vi "websocket initialization handshake.vi"(8 "error in":errorcluster, 11 "upgrade data":T1) -> (0 "error out":errorcluster, 3 "TCP Network Connection out":refnum<k5>)   [LabVIEW 2016, in "websocket upgrade handler.lvclass"]
uses:
  websocket upgrade handler.lvclass
  HTTP responder/http upgrade data.ctl
  HTTP server/http request.ctl
  HTTP server/http method.ctl
  HTTP server/http header data.ctl
  HTTP server/http response.ctl
  HTTP server/http response packet type.ctl
  HTTP server/http add header to set.vi
  HTTP server/Basic HTTP server.lvclass
  websocket core.lvlib
  HTTP server/headers/http headers.lvlib
  HTTP responder/http responder.lvclass
panel:
  out "subprotocol":string
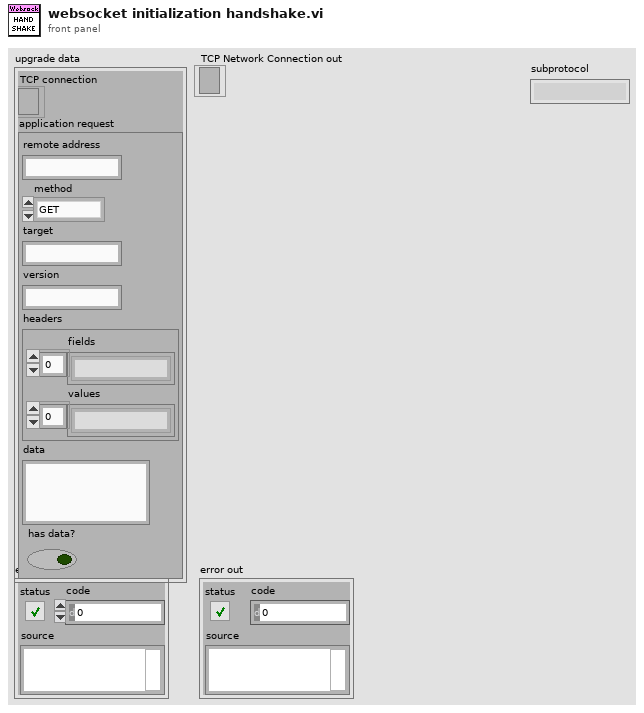
[diagram p1: front panel]
types:
  T1 = typedef "http responder.lvclass/http upgrade data.ctl" = cluster{"TCP connection":refnum<k5>, "application request":T2}
  T2 = typedef "Basic HTTP server.lvclass/http request.ctl" = cluster{"remote address":string, "method":T3, "target":string, "version":string, "headers":T4, "data":string, "has data?":bool}
  T3 = typedef "Basic HTTP server.lvclass/http method.ctl" = enum16{"GET", "POST", "PUT", "DELETE", "HEAD", "OPTIONS", "upgrade"}
  T4 = typedef "http headers.lvlib/http header data.ctl" = cluster{"fields":string[], "values":string[]}
  T5 = typedef "Basic HTTP server.lvclass/http response packet type.ctl" = enum16{"full response", "header only", "data only", "last data"}
  T6 = typedef "Basic HTTP server.lvclass/http response.ctl" = cluster{"packet type":T5, "reason code":u16, "status string":string, "headers":T4, "cookies":string[], "data":string}
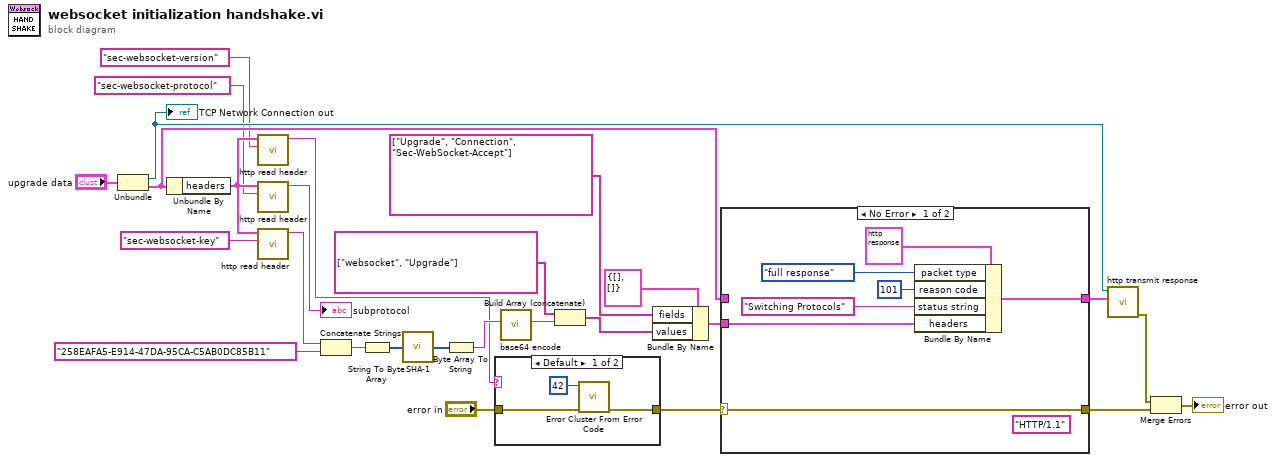
[diagram p0: block diagram]
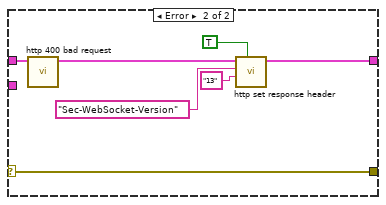
[diagram p3: hidden frame]
diagram:
  n1 = Unbundle("upgrade data") -> ("TCP connection"=w26:refnum<k5>, "application request"=w25:T2)
  "TCP Network Connection out" <- w26
  n2 = Unbundle By Name(w25) -> ("headers"=w8:T4)
  n3 = call "http read header.vi"("header field name"="sec-websocket-version" ("name"), "headers"=w8) -> ("value"=w4:string)  [unwired: 8 in, 1 out]
  n4 = call "http read header.vi"("header field name"="sec-websocket-protocol" ("name"), "headers"=w8) -> ("value"=→"subprotocol":string)  [unwired: 8 in, 1 out]
  n5 = call "http read header.vi"("header field name"="sec-websocket-key" ("name"), "headers"=w8) -> ("value"=w6:string)  [unwired: 8 in, 1 out]
  n6 = Concatenate Strings(w6, "258EAFA5-E914-47DA-95CA-C5AB0DC85B11") -> (w18:string)
  n7 = String To Byte Array(string=w18) -> (unsigned byte array=w17:u8[])
  n8 = call "SHA-1.vi"("Data"=w17) -> ("message-digest"=w16:u8[])
  n9 = Byte Array To String(unsigned byte array=w16) -> (string=w15:string)
  n10 = case shown="Default" w4 {
    tunnel: [w29 w31] -> w20
    tunnel: "error in" -> [w30 w31]
    frame Default {
      n11 = call <vilib>:"Error Cluster From Error Code.vi"("error in (no error)"=w30, "error code (0)"=42) -> ("error out"=w29:errorcluster)  [unwired: 7 in]
    }
    frame "13" {
    }
  }
  n12 = call "base64 encode.vi"("string in (not encoded)"=w15) -> ("string out (base64-encoded)"=w10:string)  [unwired: 10 in]
  n13 = Build Array (concatenate)(string[] ["websocket", "Upgrade"] ("fields"), w10) -> (w9:string[])
  n14 = Bundle By Name(cluster=T4 {"fields"=[], "values"=[]} ("headers"), "fields"=string[] ["Upgrade", "Connection", "Sec-WebSocket-Accept"], "values"=w9) -> (w13:T4)
  n15 = case shown="No Error" w20 {
    selector: w20 -> [w33 w44]
    tunnel: [w37 w40] -> w23
    tunnel: w25 -> [_ w45]
    tunnel: [w33 w44] -> w21
    tunnel: w13 -> [w32 _]
    frame No Error {
      (unwired) "HTTP/1.1" ("version")
      n16 = Bundle By Name(cluster=T6 {"packet type"=enum."full response", "reason code"=0, "status string"="", "headers"={"fields"=[], "values"=[]}, "cookies"=[], "data"=""} ("application request"), "packet type"=http_response_packet_type."full response", "reason code"=u16 101, "status string"="Switching Protocols", "headers"=w32) -> (w37:T6)
    }
    frame Error {
      n17 = call "http 400 bad request.vi"("application request in"=w45) -> ("application request out"=w41:T6)  [unwired: 10 in]
      n18 = call "http set response header.vi"("override?"=TRUE, "header field data"="13" ("name"), "header field name"="Sec-WebSocket-Version" ("name"), "application request in"=w41) -> ("application request out"=w40:T6)  [unwired: 7 in]
    }
  }
  n19 = call "http transmit response.vi"("application request"=w23, "tcp connection"=w26) -> ("error out"=w24:errorcluster)  [unwired: 9 in]
  n20 = Merge Errors(w24, w21) -> (→"error out":errorcluster)
